vi "QI_rdp_with_power.vi"(10 "Array in":dbl[](array[numeric])) -> (2 "array out":dbl[](array[numeric]))   [LabVIEW 2017]
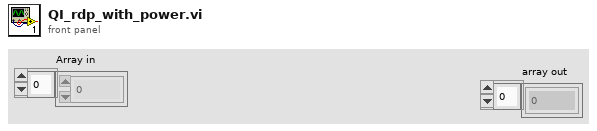
[diagram p1: front panel]
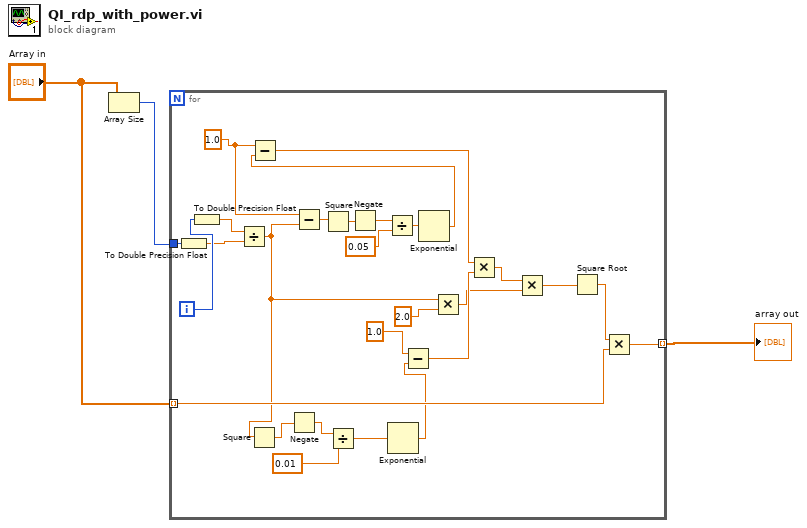
[diagram p0: block diagram]
diagram:
  n1 = Array Size(array="Array in") -> (size(s)=w3:i32)
  n2 = for {
    tunnel: w3 -> [w29]
    tunnel: "Array in" -> [w19] mode=indexing
    tunnel: [w18] -> w1 mode=indexing
    i -> [w30]
    w12 = 1.0
    n3 = To Double Precision Float(number=w29) -> (double precision float=w28:dbl)
    n4 = To Double Precision Float(number=w30) -> (double precision float=w27:dbl)
    n5 = Divide(x=w27, y=w28) -> (x/y=w11:dbl)
    n6 = Square(x=w11) -> (x^2=w14:dbl)
    n7 = Negate(x=w14) -> (-x=w13:dbl)
    n8 = Subtract(x=w12, y=w11) -> (x-y=w10:dbl)
    n9 = Square(x=w10) -> (x^2=w9:dbl)
    n10 = Divide(x=w13, y=0.01) -> (x/y=w16:dbl)
    n11 = Negate(x=w9) -> (-x=w8:dbl)
    n12 = Divide(x=w8, y=0.05) -> (x/y=w6:dbl)
    n13 = Exponential(1:w16) -> (0:w15:dbl)
    n14 = Subtract(x=1.0, y=w15) -> (x-y=w24:dbl)
    n15 = Exponential(1:w6) -> (0:w5:dbl)
    n16 = Subtract(x=w12, y=w5) -> (x-y=w25:dbl)
    n17 = Multiply(x=w11, y=2.0) -> (x*y=w22:dbl)
    n18 = Multiply(x=w25, y=w24) -> (x*y=w23:dbl)
    n19 = Multiply(x=w23, y=w22) -> (x*y=w21:dbl)
    n20 = Square Root(x=w21) -> (sqrt(x)=w20:dbl)
    n21 = Multiply(x=w20, y=w19) -> (x*y=w18:dbl)
  }
  "array out" <- w1
